vi "loadHTUPH.vi"(10 "machine":string="QAMT50") -> ()   [LabVIEW 2012]
uses:
  <vilib>/addons/database/Connection.llb/DB Tools Open Connec (Path).vi
  <vilib>/Utility/file.llb/Read From Spreadsheet File (string).vi
  <vilib>/addons/database/NI_Database_API.lvlib
panel:
  out "output cluster":T1
  out "SQL TIME":string
  out "error out":errorcluster
  in  "Cluster":T1
  out "String 12":string
  out "String 11":string
  out "after substring 14":string
  out "String 10":string
  out "after substring 13":string
  out "String 9":string
  out "String 8":string
  out "String 7":string
  out "after substring 12":string
  out "String 6":string
  out "String 5":string
  out "after substring 11":string
  out "String 4":string
  out "String 3":string
  out "after substring 10":string
  out "String 2":string
  out "String":string
  out "after substring 9":string
  out "after substring 8":string
  out "after substring 7":string
  out "after substring 6":string
  out "after substring 5":string
  out "after substring 4":string
  out "after substring 3":string
  out "after substring 2":string
  out "after substring":string
  out "all rows":string[][](array[string])
  out "filenames":string[](array[string])
  in  "base path":path=path "c:/temp/ht2000"
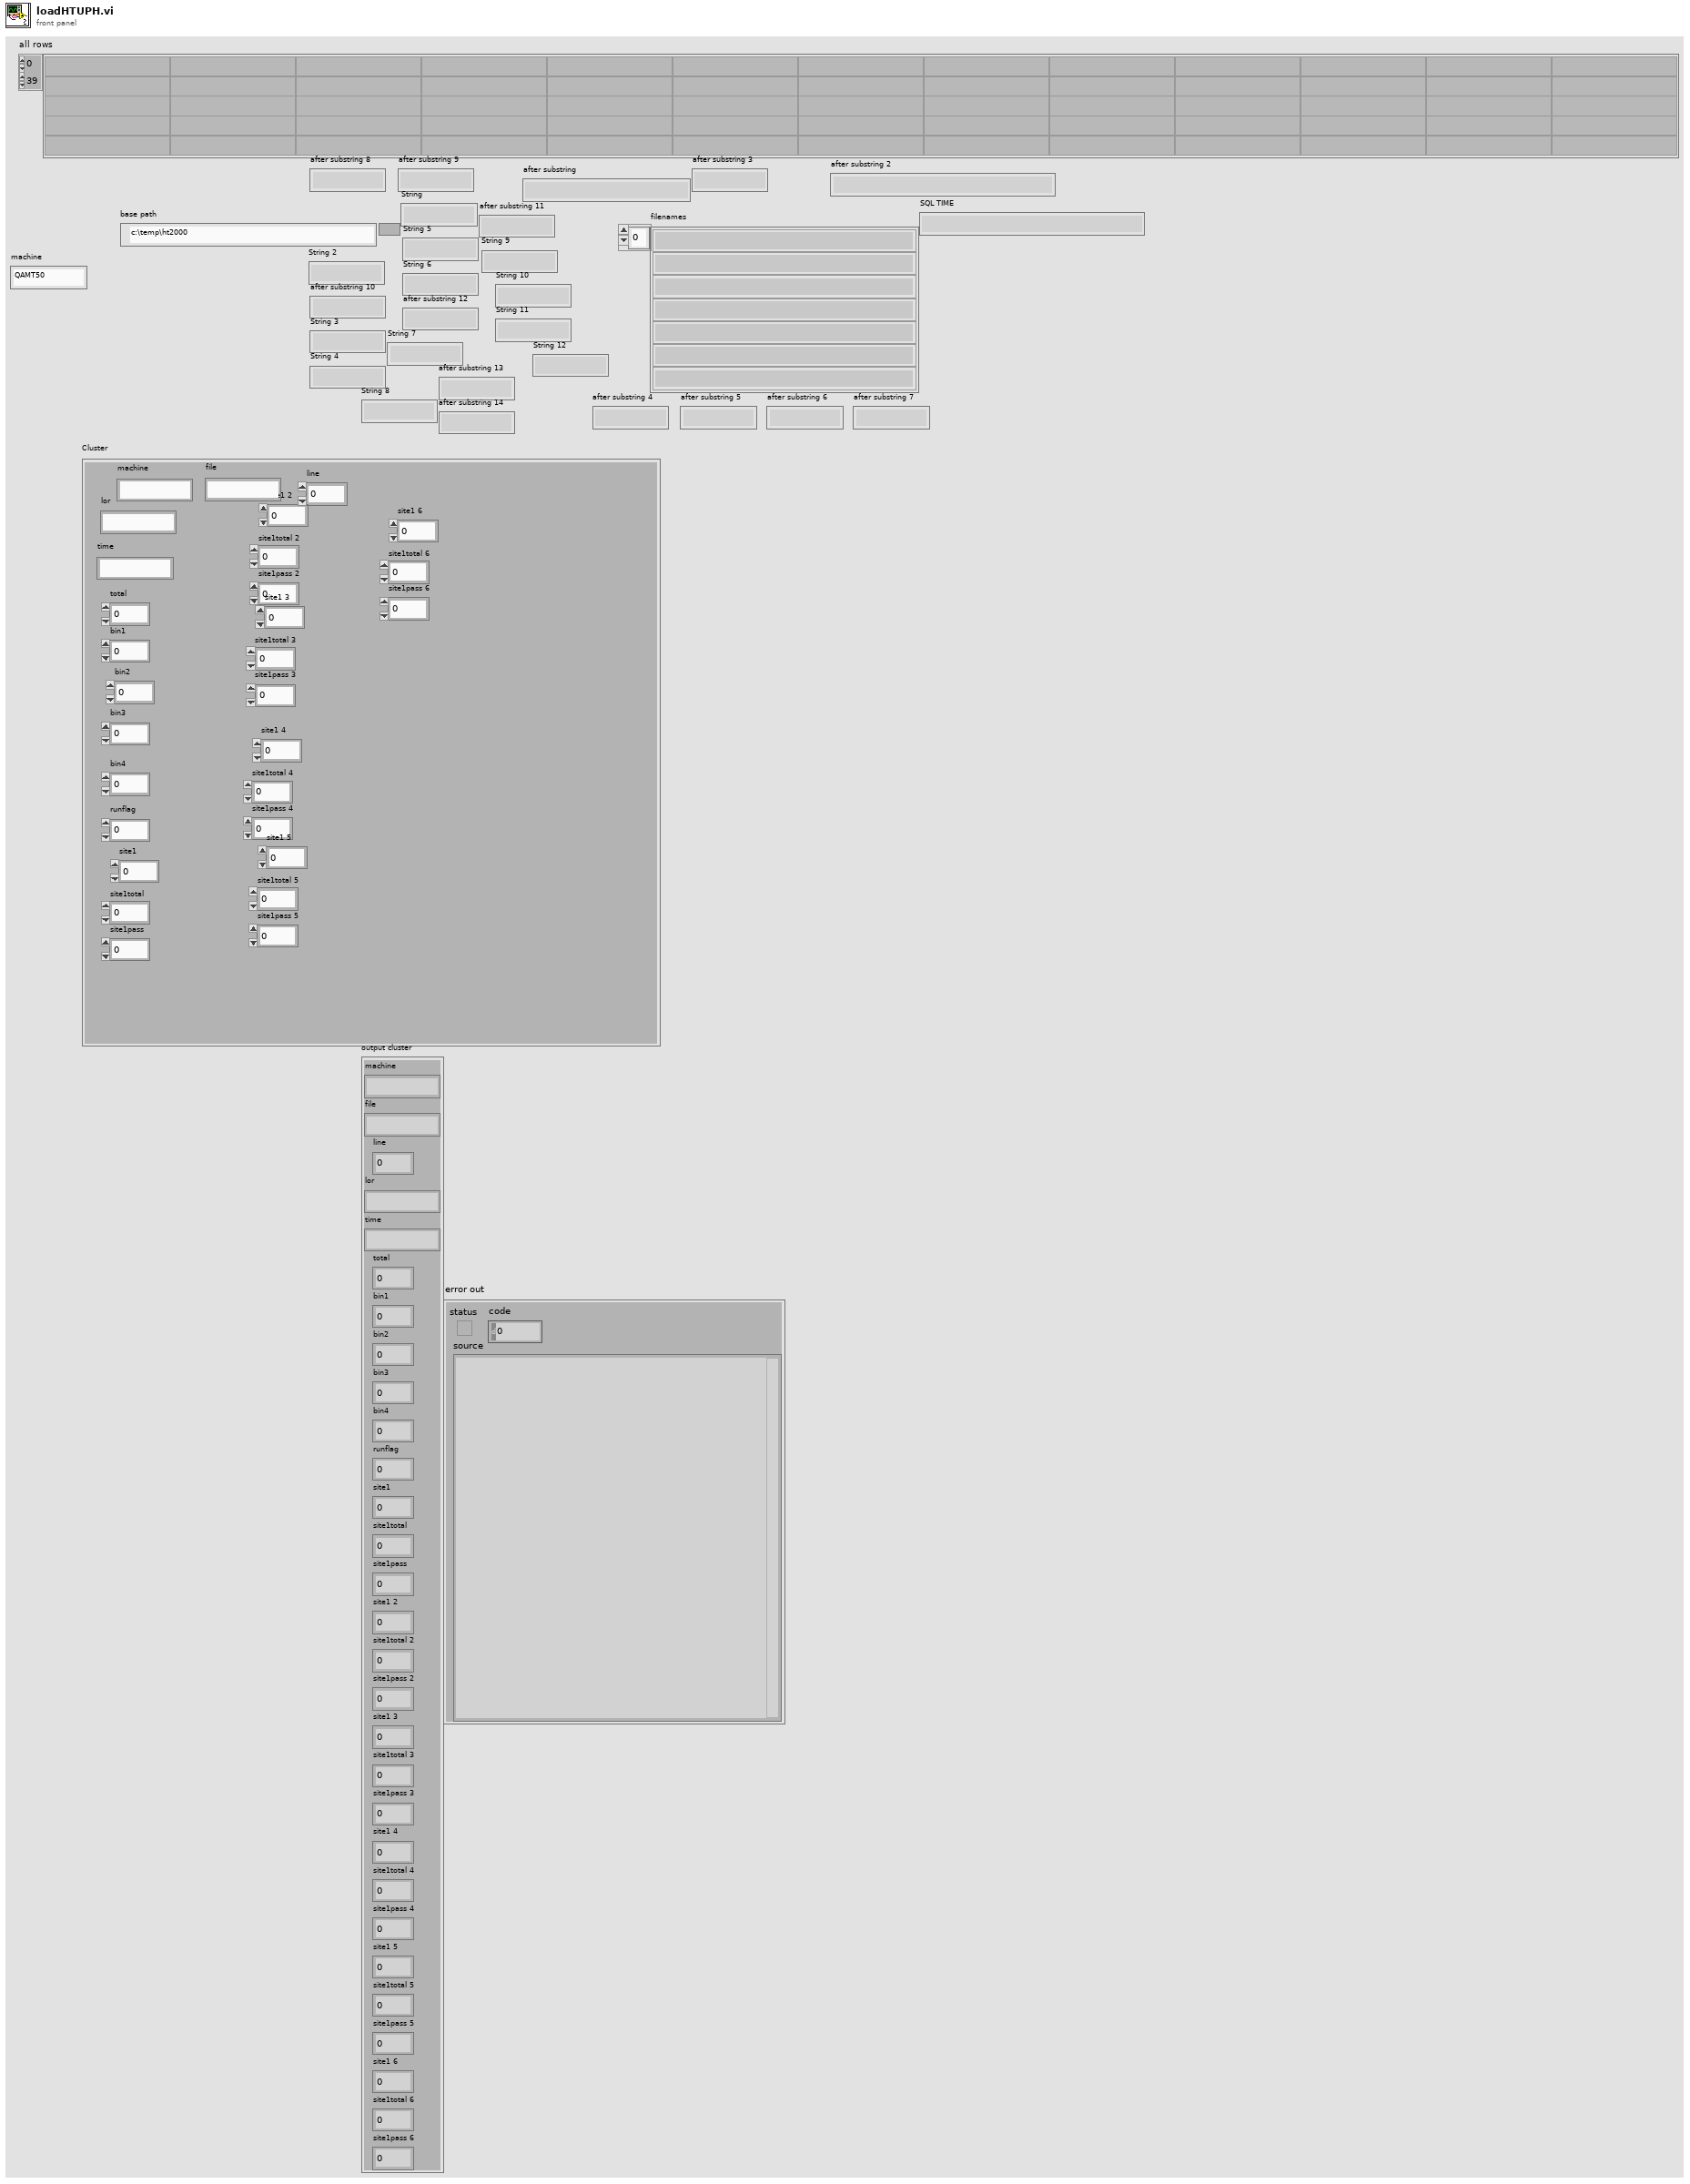
[diagram p1: front panel]
types:
  T1 = cluster{"machine":string, "file":string, "line":dbl, "lor":string, "time":string, "total":dbl, "bin1":dbl, "bin2":dbl, "bin3":dbl, "bin4":dbl, "runflag":dbl, "site1":dbl, "site1total":dbl, "site1pass":dbl, "site1 2":dbl, "site1total 2":dbl, "site1pass 2":dbl, "site1 3":dbl, "site1total 3":dbl, "site1pass 3":dbl, "site1 4":dbl, "site1total 4":dbl, "site1pass 4":dbl, "site1 5":dbl, "site1total 5":dbl, "site1pass 5":dbl, "site1 6":dbl, "site1total 6":dbl, "site1pass 6":dbl}
  T2 = typedef "NI_Database_API.lvlib/Conn ObjectReference.ctl" = refnum<k1>
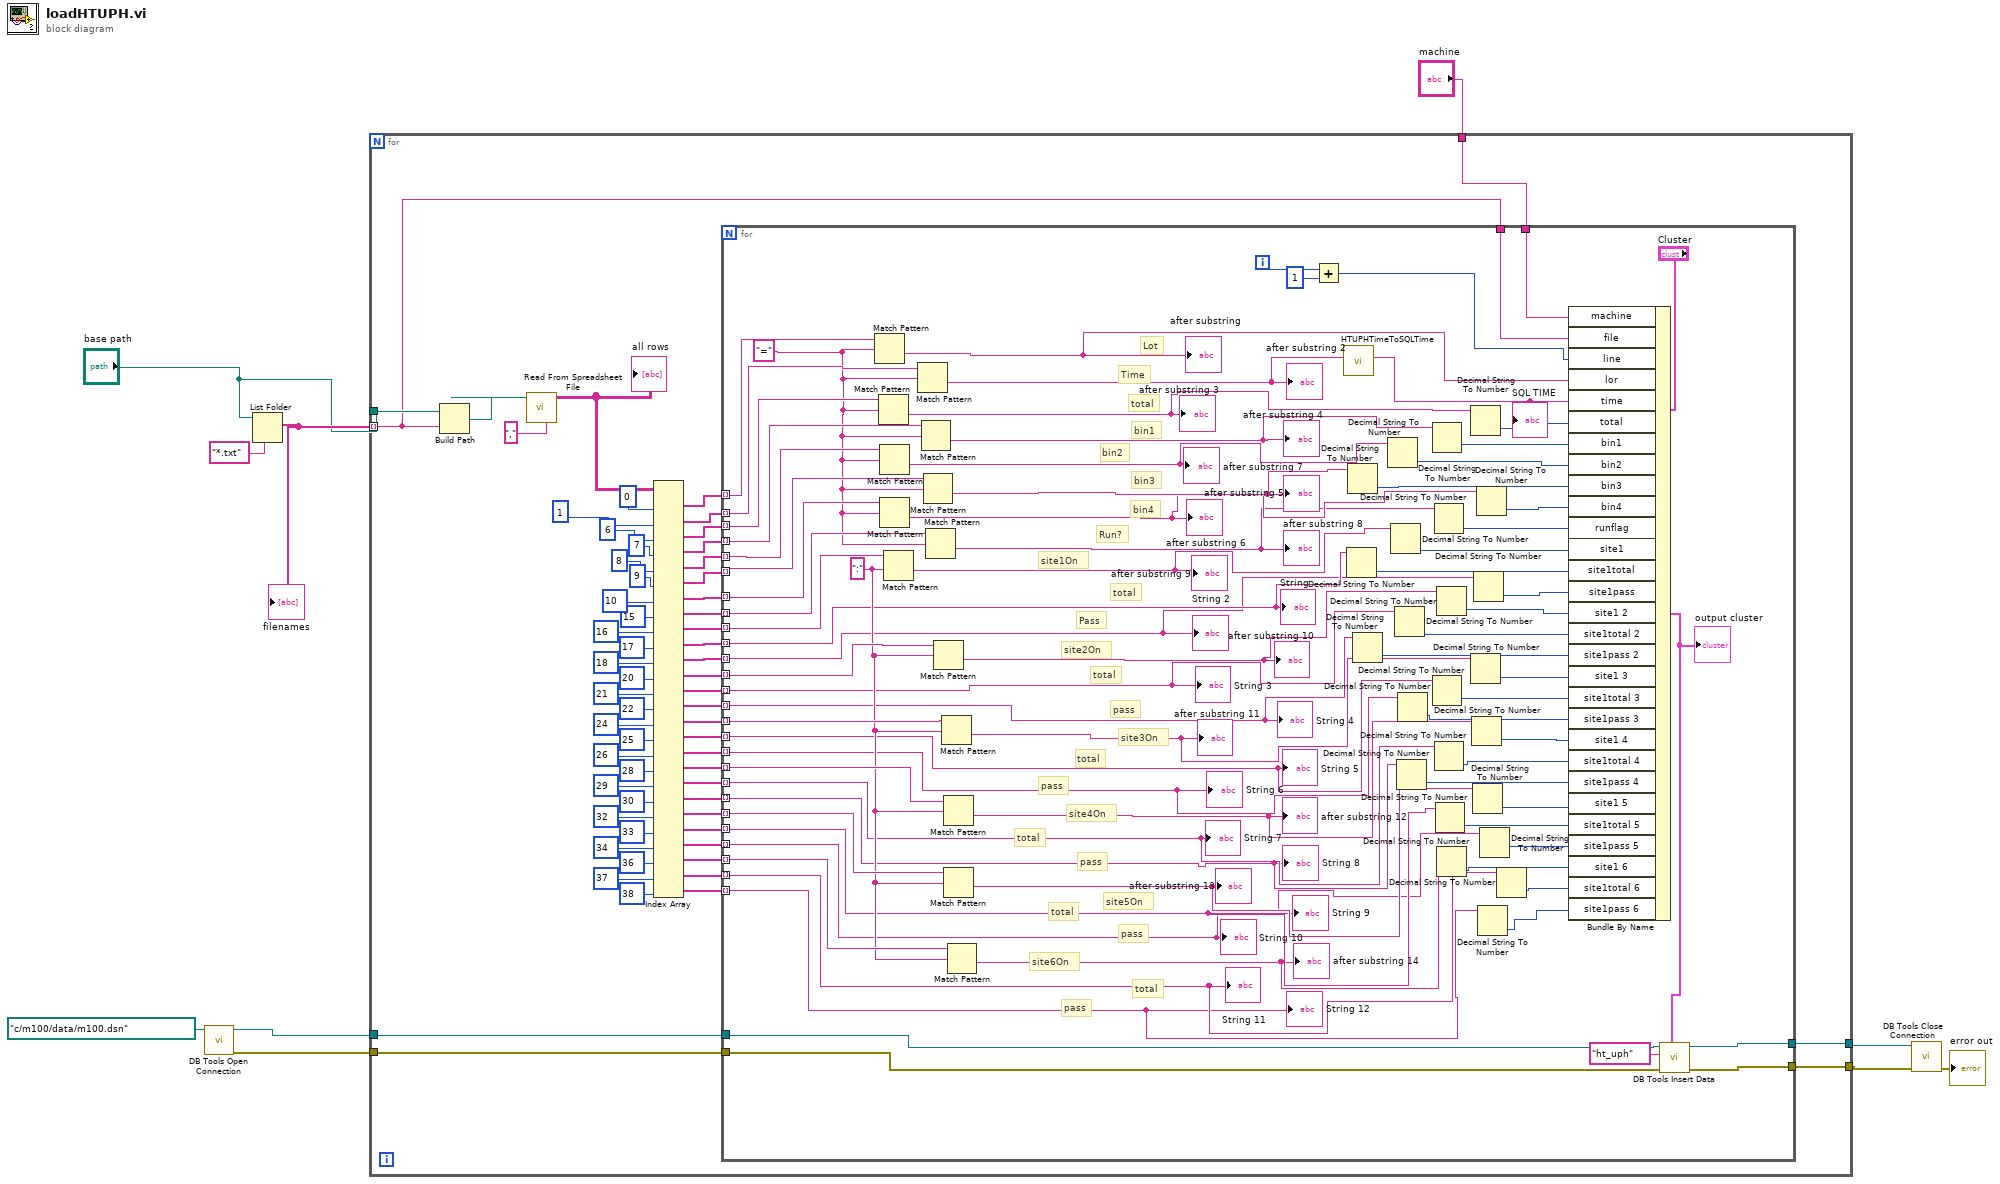
[diagram p0: block diagram]
diagram:
  n1 = call-poly <vilib>:"DB Tools Open Connection.vi"("connection information"=path "c:/m100/data/m100.dsn") -> ("error out"=w5:errorcluster, "connection reference"=w6:T2)  [unwired: 7 in]
  n2 = List Folder(path="base path", pattern="*.txt") -> (filenames=w9:string[])  [unwired: 2 in, 3 out]
  "filenames" <- w9
  n3 = for {
    tunnel: w9 -> [w11] mode=indexing
    tunnel: "base path" -> [w70]
    tunnel: w6 -> [w16]
    tunnel: w5 -> [w15]
    tunnel: [w14] -> w4
    tunnel: [w13] -> w3
    tunnel: "machine" -> [w12]
    n4 = Build Path(base path=w70, name or relative path=w11) -> (appended path=w71:path)
    n5 = call-poly <vilib>:"Read From Spreadsheet File.vi"("delimiter (\\t)"="," ("delimiter (\\t)"), "file path (dialog if empty)"=w71) -> ("all rows"=w69:string[][])  [unwired: 5 in, 4 out]
    "all rows" <- w69
    n6 = Index Array(array=w69, index (col) #1=0 ("index (row)"), index (col) #2=1 ("disabled index (col)"), index (col) #3=6 ("index (col)"), index (col) #4=7 ("index (col)"), index (col) #5=8 ("index (col)"), index (col) #6=9 ("index (col)"), index (col) #7=10 ("index (col)"), index (col) #8=15 ("index (col)"), index (col) #9=16 ("index (col)"), index (col) #10=17 ("index (col)"), index (col) #11=18 ("index (col)"), index (col) #12=20 ("index (col)"), index (col) #13=21 ("index (col)"), index (col) #14=22 ("index (col)"), index (col) #15=24 ("index (col)"), index (col) #16=25 ("index (col)"), index (col) #17=26 ("index (col)"), index (col) #18=28 ("index (col)"), index (col) #19=29 ("index (col)"), index (col) #20=30 ("index (col)"), index (col) #21=32 ("index (col)"), index (col) #22=33 ("index (col)"), index (col) #23=34 ("index (col)"), index (col) #24=36 ("index (col)"), index (col) #25=37 ("index (col)"), index (col) #26=38 ("index (col)")) -> (element #1=w67:string[], element #2=w66:string[], element #3=w63:string[], element #4=w58:string[], element #5=w57:string[], element #6=w56:string[], element #7=w55:string[], element #8=w50:string[], element #9=w49:string[], element #10=w48:string[], element #11=w47:string[], element #12=w43:string[], element #13=w42:string[], element #14=w41:string[], element #15=w37:string[], element #16=w36:string[], element #17=w35:string[], element #18=w31:string[], element #19=w30:string[], element #20=w29:string[], element #21=w22:string[], element #22=w21:string[], element #23=w20:string[], element #24=w19:string[], element #25=w18:string[], element #26=w17:string[])  [unwired: 26 in]
    n7 = for {
      tunnel: w67 -> [w151] mode=indexing
      tunnel: w66 -> [w144] mode=indexing
      tunnel: w63 -> [w150] mode=indexing
      tunnel: w58 -> [w149] mode=indexing
      tunnel: w57 -> [w148] mode=indexing
      tunnel: w56 -> [w147] mode=indexing
      tunnel: w55 -> [w146] mode=indexing
      tunnel: w50 -> [w145] mode=indexing
      tunnel: w49 -> [w143] mode=indexing
      tunnel: w48 -> [w116] mode=indexing
      tunnel: w47 -> [w114] mode=indexing
      tunnel: w43 -> [w141] mode=indexing
      tunnel: w42 -> [w110] mode=indexing
      tunnel: w41 -> [w108] mode=indexing
      tunnel: w37 -> [w140] mode=indexing
      tunnel: w36 -> [w104] mode=indexing
      tunnel: w35 -> [w102] mode=indexing
      tunnel: w31 -> [w139] mode=indexing
      tunnel: w30 -> [w98] mode=indexing
      tunnel: w29 -> [w96] mode=indexing
      tunnel: w22 -> [w138] mode=indexing
      tunnel: w21 -> [w92] mode=indexing
      tunnel: w20 -> [w90] mode=indexing
      tunnel: w19 -> [w137] mode=indexing
      tunnel: w18 -> [w86] mode=indexing
      tunnel: w17 -> [w84] mode=indexing
      tunnel: w16 -> [w83]
      tunnel: w15 -> [w82]
      tunnel: [w81] -> w14
      tunnel: [w80] -> w13
      tunnel: w12 -> [w77]
      tunnel: w11 -> [w76]
      i -> [w75]
      w136 = ":" ("regular expression")
      w142 = "=" ("regular expression")
      # "pass"
      # "total"
      # "site6On"
      # "pass"
      # "total"
      # "site5On"
      # "pass"
      # "total"
      # "site4On"
      # "pass"
      # "total"
      # "site3On"
      # "pass"
      # "total"
      # "site2On"
      # "Pass"
      # "total"
      # "site1On"
      # "Run?"
      # "bin4"
      # "bin3"
      # "bin2"
      # "bin1"
      # "total"
      # "Time"
      # "Lot"
      n8 = Match Pattern(string=w151, regular expression=w142) -> (after substring=w134:string)  [unwired: 1 in, 3 out]
      "after substring" <- w134
      n9 = Match Pattern(string=w150, regular expression=w142) -> (after substring=w131:string)  [unwired: 1 in, 3 out]
      "after substring 3" <- w131
      n10 = Match Pattern(string=w148, regular expression=w142) -> (after substring=w126:string)  [unwired: 1 in, 3 out]
      "after substring 7" <- w126
      n11 = Match Pattern(string=w146, regular expression=w142) -> (after substring=w122:string)  [unwired: 1 in, 3 out]
      "after substring 6" <- w122
      n12 = Match Pattern(string=w143, regular expression=w136) -> (after substring=w118:string)  [unwired: 1 in, 3 out]
      "after substring 9" <- w118
      n13 = Match Pattern(string=w144, regular expression=w142) -> (after substring=w133:string)  [unwired: 1 in, 3 out]
      "after substring 2" <- w133
      n14 = Match Pattern(string=w149, regular expression=w142) -> (after substring=w128:string)  [unwired: 1 in, 3 out]
      "after substring 4" <- w128
      n15 = Match Pattern(string=w147, regular expression=w142) -> (after substring=w124:string)  [unwired: 1 in, 3 out]
      "after substring 5" <- w124
      n16 = Match Pattern(string=w145, regular expression=w142) -> (after substring=w120:string)  [unwired: 1 in, 3 out]
      "after substring 8" <- w120
      n17 = Match Pattern(string=w141, regular expression=w136) -> (after substring=w112:string)  [unwired: 1 in, 3 out]
      "after substring 10" <- w112
      n18 = Match Pattern(string=w140, regular expression=w136) -> (after substring=w106:string)  [unwired: 1 in, 3 out]
      "after substring 11" <- w106
      n19 = Match Pattern(string=w139, regular expression=w136) -> (after substring=w100:string)  [unwired: 1 in, 3 out]
      "after substring 12" <- w100
      n20 = Match Pattern(string=w138, regular expression=w136) -> (after substring=w94:string)  [unwired: 1 in, 3 out]
      "after substring 13" <- w94
      n21 = Match Pattern(string=w137, regular expression=w136) -> (after substring=w88:string)  [unwired: 1 in, 3 out]
      "after substring 14" <- w88
      n22 = Add(x=w75, y=1) -> (x+y=w73:i32)
      n23 = call "HTUPHTimeToSQLTime.vi"("UPHTime"=w133) -> ("SQL TIME"=w132:string)  [unwired: 10 in]
      "SQL TIME" <- w132
      n24 = Decimal String To Number(string=w116) -> (number=w117:i32)  [unwired: 2 in, 1 out]
      n25 = Decimal String To Number(string=w124) -> (number=w125:i32)  [unwired: 2 in, 1 out]
      n26 = Decimal String To Number(string=w108) -> (number=w109:i32)  [unwired: 2 in, 1 out]
      n27 = Decimal String To Number(string=w126) -> (number=w127:i32)  [unwired: 2 in, 1 out]
      n28 = Decimal String To Number(string=w118) -> (number=w119:i32)  [unwired: 2 in, 1 out]
      n29 = Decimal String To Number(string=w110) -> (number=w111:i32)  [unwired: 2 in, 1 out]
      n30 = Decimal String To Number(string=w96) -> (number=w97:i32)  [unwired: 2 in, 1 out]
      n31 = Decimal String To Number(string=w102) -> (number=w103:i32)  [unwired: 2 in, 1 out]
      n32 = Decimal String To Number(string=w128) -> (number=w129:i32)  [unwired: 2 in, 1 out]
      n33 = Decimal String To Number(string=w104) -> (number=w105:i32)  [unwired: 2 in, 1 out]
      n34 = Decimal String To Number(string=w120) -> (number=w121:i32)  [unwired: 2 in, 1 out]
      n35 = Decimal String To Number(string=w98) -> (number=w99:i32)  [unwired: 2 in, 1 out]
      n36 = Decimal String To Number(string=w92) -> (number=w93:i32)  [unwired: 2 in, 1 out]
      n37 = Decimal String To Number(string=w112) -> (number=w113:i32)  [unwired: 2 in, 1 out]
      n38 = Decimal String To Number(string=w88) -> (number=w89:i32)  [unwired: 2 in, 1 out]
      n39 = Decimal String To Number(string=w131) -> (number=w130:i32)  [unwired: 2 in, 1 out]
      n40 = Decimal String To Number(string=w106) -> (number=w107:i32)  [unwired: 2 in, 1 out]
      n41 = Decimal String To Number(string=w100) -> (number=w101:i32)  [unwired: 2 in, 1 out]
      n42 = Decimal String To Number(string=w94) -> (number=w95:i32)  [unwired: 2 in, 1 out]
      n43 = Decimal String To Number(string=w114) -> (number=w115:i32)  [unwired: 2 in, 1 out]
      n44 = Decimal String To Number(string=w122) -> (number=w123:i32)  [unwired: 2 in, 1 out]
      n45 = Decimal String To Number(string=w84) -> (number=w85:i32)  [unwired: 2 in, 1 out]
      n46 = Decimal String To Number(string=w90) -> (number=w91:i32)  [unwired: 2 in, 1 out]
      n47 = Decimal String To Number(string=w86) -> (number=w87:i32)  [unwired: 2 in, 1 out]
      n48 = Bundle By Name(cluster="Cluster", "machine"=w77, "file"=w76, "line"=w73, "lor"=w134, "time"=w132, "total"=w130, "bin1"=w129, "bin2"=w127, "bin3"=w125, "bin4"=w123, "runflag"=w121, "site1"=w119, "site1total"=w117, "site1pass"=w115, "site1 2"=w113, "site1total 2"=w111, "site1pass 2"=w109, "site1 3"=w107, "site1total 3"=w105, "site1pass 3"=w103, "site1 4"=w101, "site1total 4"=w99, "site1pass 4"=w97, "site1 5"=w95, "site1total 5"=w93, "site1pass 5"=w91, "site1 6"=w89, "site1total 6"=w87, "site1pass 6"=w85) -> (w78:T1)
      "output cluster" <- w78
      n49 = call <vilib>:"DB Tools Insert Data.vi"("data"=w78, "error in (no error)"=w82, "table"="ht_uph", "connection reference"=w83) -> ("error out"=w80:errorcluster, "connection reference out"=w81:T2)  [unwired: 6 in]
      "String" <- w116
      "String 2" <- w114
      "String 3" <- w110
      "String 4" <- w108
      "String 5" <- w104
      "String 6" <- w102
      "String 7" <- w98
      "String 8" <- w96
      "String 9" <- w92
      "String 10" <- w90
      "String 11" <- w86
      "String 12" <- w84
    }
  }
  n50 = call <vilib>:"DB Tools Close Connection.vi"("error in (no error)"=w3, "connection reference"=w4) -> ("error out"=→"error out":errorcluster)  [unwired: 5 in]
